vi "To String Array.vi"(8 "error in (no error)":errorcluster, 11 "Wait On Boolean Config in":refnum<class "Wait On Boolean Step Config.lvclass">) -> (0 "error out":errorcluster, 1 "Step String Array":string[](array[string]), 3 "Wait On Boolean Config out":refnum<class "Wait On Boolean Step Config.lvclass">)   [LabVIEW 2018, in "Wait On Boolean Step Config.lvclass"]
uses:
  Wait On Boolean Step Config.lvclass
  Wait On Boolean Step Config.lvclass/Wait On Boolean Step Config.ctl
  <vilib>/NI/Tag Bus/tag/tag descriptor.lvclass/tag descriptor.ctl
  <vilib>/NI/Tag Bus Module Framework/channel/TBM channel.lvclass
  C:/Program Files (x86)/National Instruments/LabVIEW 2018/vi.lib/NI/Tag Bus/tag/tag descriptor.lvclass
  classes/Step/Config/Step Config.lvclass
  <vilib>/NI/Tag Bus/tag/tag descriptor.lvclass
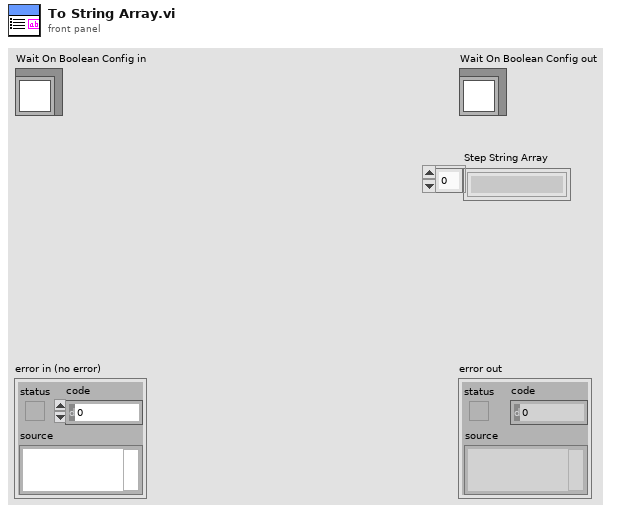
[diagram p1: front panel]
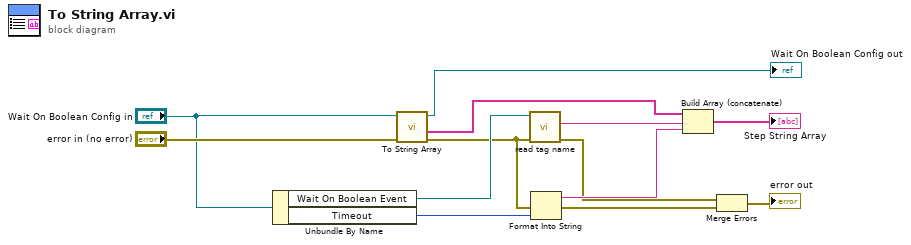
[diagram p0: block diagram]
diagram:
  n1 = Unbundle By Name("Wait On Boolean Config in") -> ("Wait On Boolean Event"=w10:refnum<class "TBM channel.lvclass">, "Timeout"=w9:i32)
  n2 = call-parent "To String Array.vi"("error in (no error)"="error in (no error)", "Step Config in"="Wait On Boolean Config in") -> ("error out"=w5:errorcluster, "Step String Array"=w8:string[], "Step Config out"=→"Wait On Boolean Config out":refnum<class "Wait On Boolean Step Config.lvclass">)  [unwired: 7 in]
  n3 = call <vilib>:"read tag name.vi"("error in"=w5, "system tag in"=w10) -> ("error out"=w3:errorcluster, "name"=w6:string)  [unwired: 7 in, 1 out]
  n4 = Format Into String(error in=w5, w9) -> (resulting string=w7:string, error out=w4:errorcluster)  [unwired: 2 in]
  n5 = Build Array (concatenate)(w8, w6, w7) -> (→"Step String Array":string[])
  n6 = Merge Errors(w3, w4) -> (→"error out":errorcluster)
